vi "MotorControllerGUI.vi"() -> ()   [LabVIEW 2017]
uses:
  device_list.ctl
  device.ctl
  location.ctl
  Newport.CONEXCC.CommandInterface
  <vilib>/Utility/miscctls.llb/LVAnnotationListTypeDef.ctl
  <vilib>/lvdsc/NI_DSC.lvlib
panel:
  out "String":string
  out "Numeric":i32
  in  "Home Y?":bool
  in  "Home X?":bool
  in  "Y COM port":refnum<visa-resource-name>="COM3"
  in  "X COM port":refnum<visa-resource-name>="COM4"
  out "Boolean":bool
  out "error out 2":errorcluster
  in  "Direction Pad":T1={"right+"=FALSE, "right"=FALSE, "left"=FALSE, "left+"=FALSE, "up"=FALSE, "up+"=FALSE, "down+"=FALSE, "down"=FALSE, "motor stop"=FALSE, "Velocity (mm/s)"=2.0, "Step (mm)"=0.1}
  out "Current Location":T2 {"Position"."Position Y" format="%#.3f"; "Position"."Position X" format="%#.3f"}
  out "Key Move?":bool
  out "Center location":T2 {"Position"."Position Y" format="%#.3f"; "Position"."Position X" format="%#.3f"}
  out "Circle":cluster{dbl[], dbl[]}
  in  "Location Description":string="Center"
  in  "Device Description":string="Layout"
  in  "Radius Limit (mm)":dbl=5.0
  out "PA_Set 2":i32
  out "PA_Set":i32
  out "errstring 2":string
  out "errstring":string
  out "error out":errorcluster
  out "X Motor ID":string
  out "Y Motor ID":string
  in  "Delete device":bool
  in  "Device":u16(ring) items=["Layout", "AutoTetherSaver"]
  out "Mouse over item?":bool
  out "Mouse over location":cluster{"X":dbl, "Y":dbl}
  in  "List of default devices":T3 {"List of locations"."Position"."Position Y" format="%#.3f"; "List of locations"."Position"."Position X" format="%#.3f"}
  in  "Load device list":bool
  in  "Default File Path":path
  in  "Add location":bool
  out "Last click location":cluster{"X":dbl, "Y":dbl}
  in  "Rescale location plot":bool caption="Rescale"
  out "Goto Location":T2 {"Position"."Position Y" format="%#.3f"; "Position"."Position X" format="%#.3f"}
  in  "Save device list":bool
  in  "List of devices":T3 {"List of locations"."Position"."Position Y" format="%#.3f"; "List of locations"."Position"."Position X" format="%#.3f"}
  in  "stop":bool
  in  "nSWAT quick move diagram":T5
  out "Location plot":cluster{dbl[], dbl[]}[](graph)
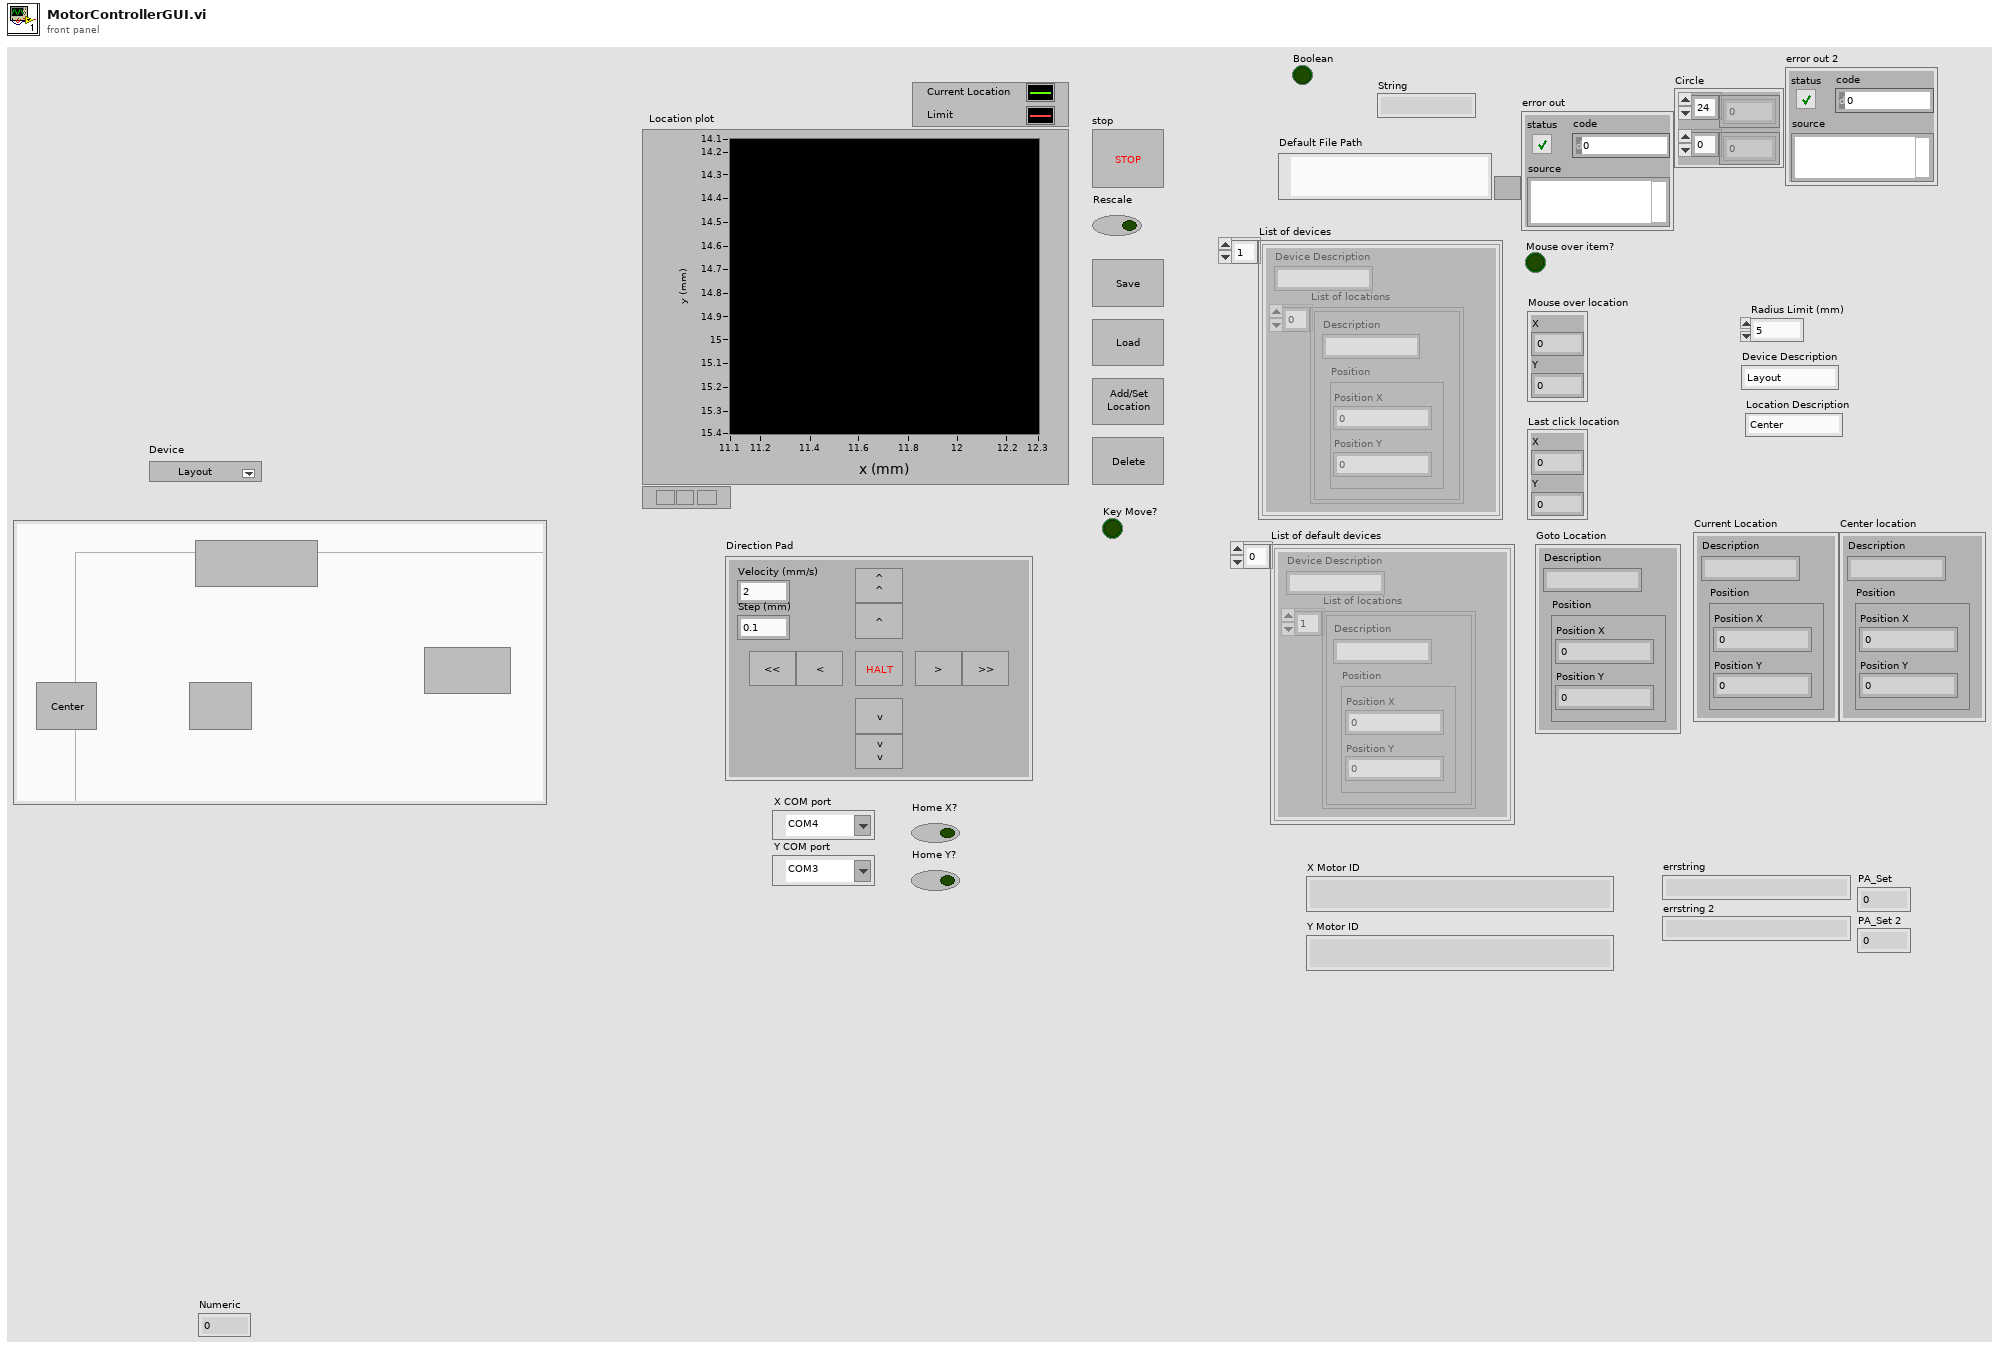
[diagram p1: front panel]
types:
  T1 = cluster{"right+":bool, "right":bool, "left":bool, "left+":bool, "up":bool, "up+":bool, "down+":bool, "down":bool, "motor stop":bool, "Velocity (mm/s)":dbl, "Step (mm)":dbl}
  T2 = typedef "location.ctl" = cluster{"Description":string, "Position":cluster{"Position X":dbl, "Position Y":dbl}}
  T3 = typedef "device_list.ctl" = T4[]
  T4 = typedef "device.ctl" = cluster{"List of locations":T2[], "Device Description":string}
  T5 = cluster{"Button 0":bool, "Button 1":bool, "Button 2":bool, "Button 3":bool}
  T6 = typedef "eventvkey.ctl" = enum16{"ASCII", "Enter", "Return", "Shift", "Ctrl", "Alt", "Cmd", "Opt", "Caps", "NumLock", "Clear", "Break", "Up", "Down", "Left", "Right", "Insert", "Delete", "Home", "End", "PageUp", "PageDown", "Escape", "Help", "Pause", "ScrollLock", "F1", "F2", "F3", "F4", "F5", "F6", "F7", "F8", "F9", "F10", "F11", "F12", "F13", "F14", "F15", "F16", "F17", "F18", "F19", "F20", "F21", "F22", "F23", "F24", "Play", "VolumeUp", "VolumeDown", "Mute", "Two Byte Char"}
  T7 = typedef "LVAnnotationListTypeDef.ctl" = cluster{"Name":string, "Color":u32, "Style":u8, "Point Style":u8, "Name Visible":bool, "Allow Drag":bool, "Annotation Mode":u32, "Plot":i32, "Index":i32, "Position":cluster{"X":dbl, "Y":dbl}, "X Scale":u32, "Y Scale":u32, "Show Arrow":bool, "Lock Name":bool, "Plot Area":i32, "Label Offset":cluster{"X":dbl, "Y":dbl}}[]
  T8 = cluster{"Name":string, "Color":u32, "Style":u8, "Point Style":u8, "Name Visible":bool, "Allow Drag":bool, "Annotation Mode":u32, "Plot":i32, "Index":i32, "Position":cluster{"X":dbl, "Y":dbl}, "X Scale":u32, "Y Scale":u32, "Show Arrow":bool, "Lock Name":bool, "Plot Area":i32, "Label Offset":cluster{"X":dbl, "Y":dbl}}
  T9 = typedef "LVPoint32TypeDef.ctl" = cluster{"Horizontal":i32, "Vertical":i32}
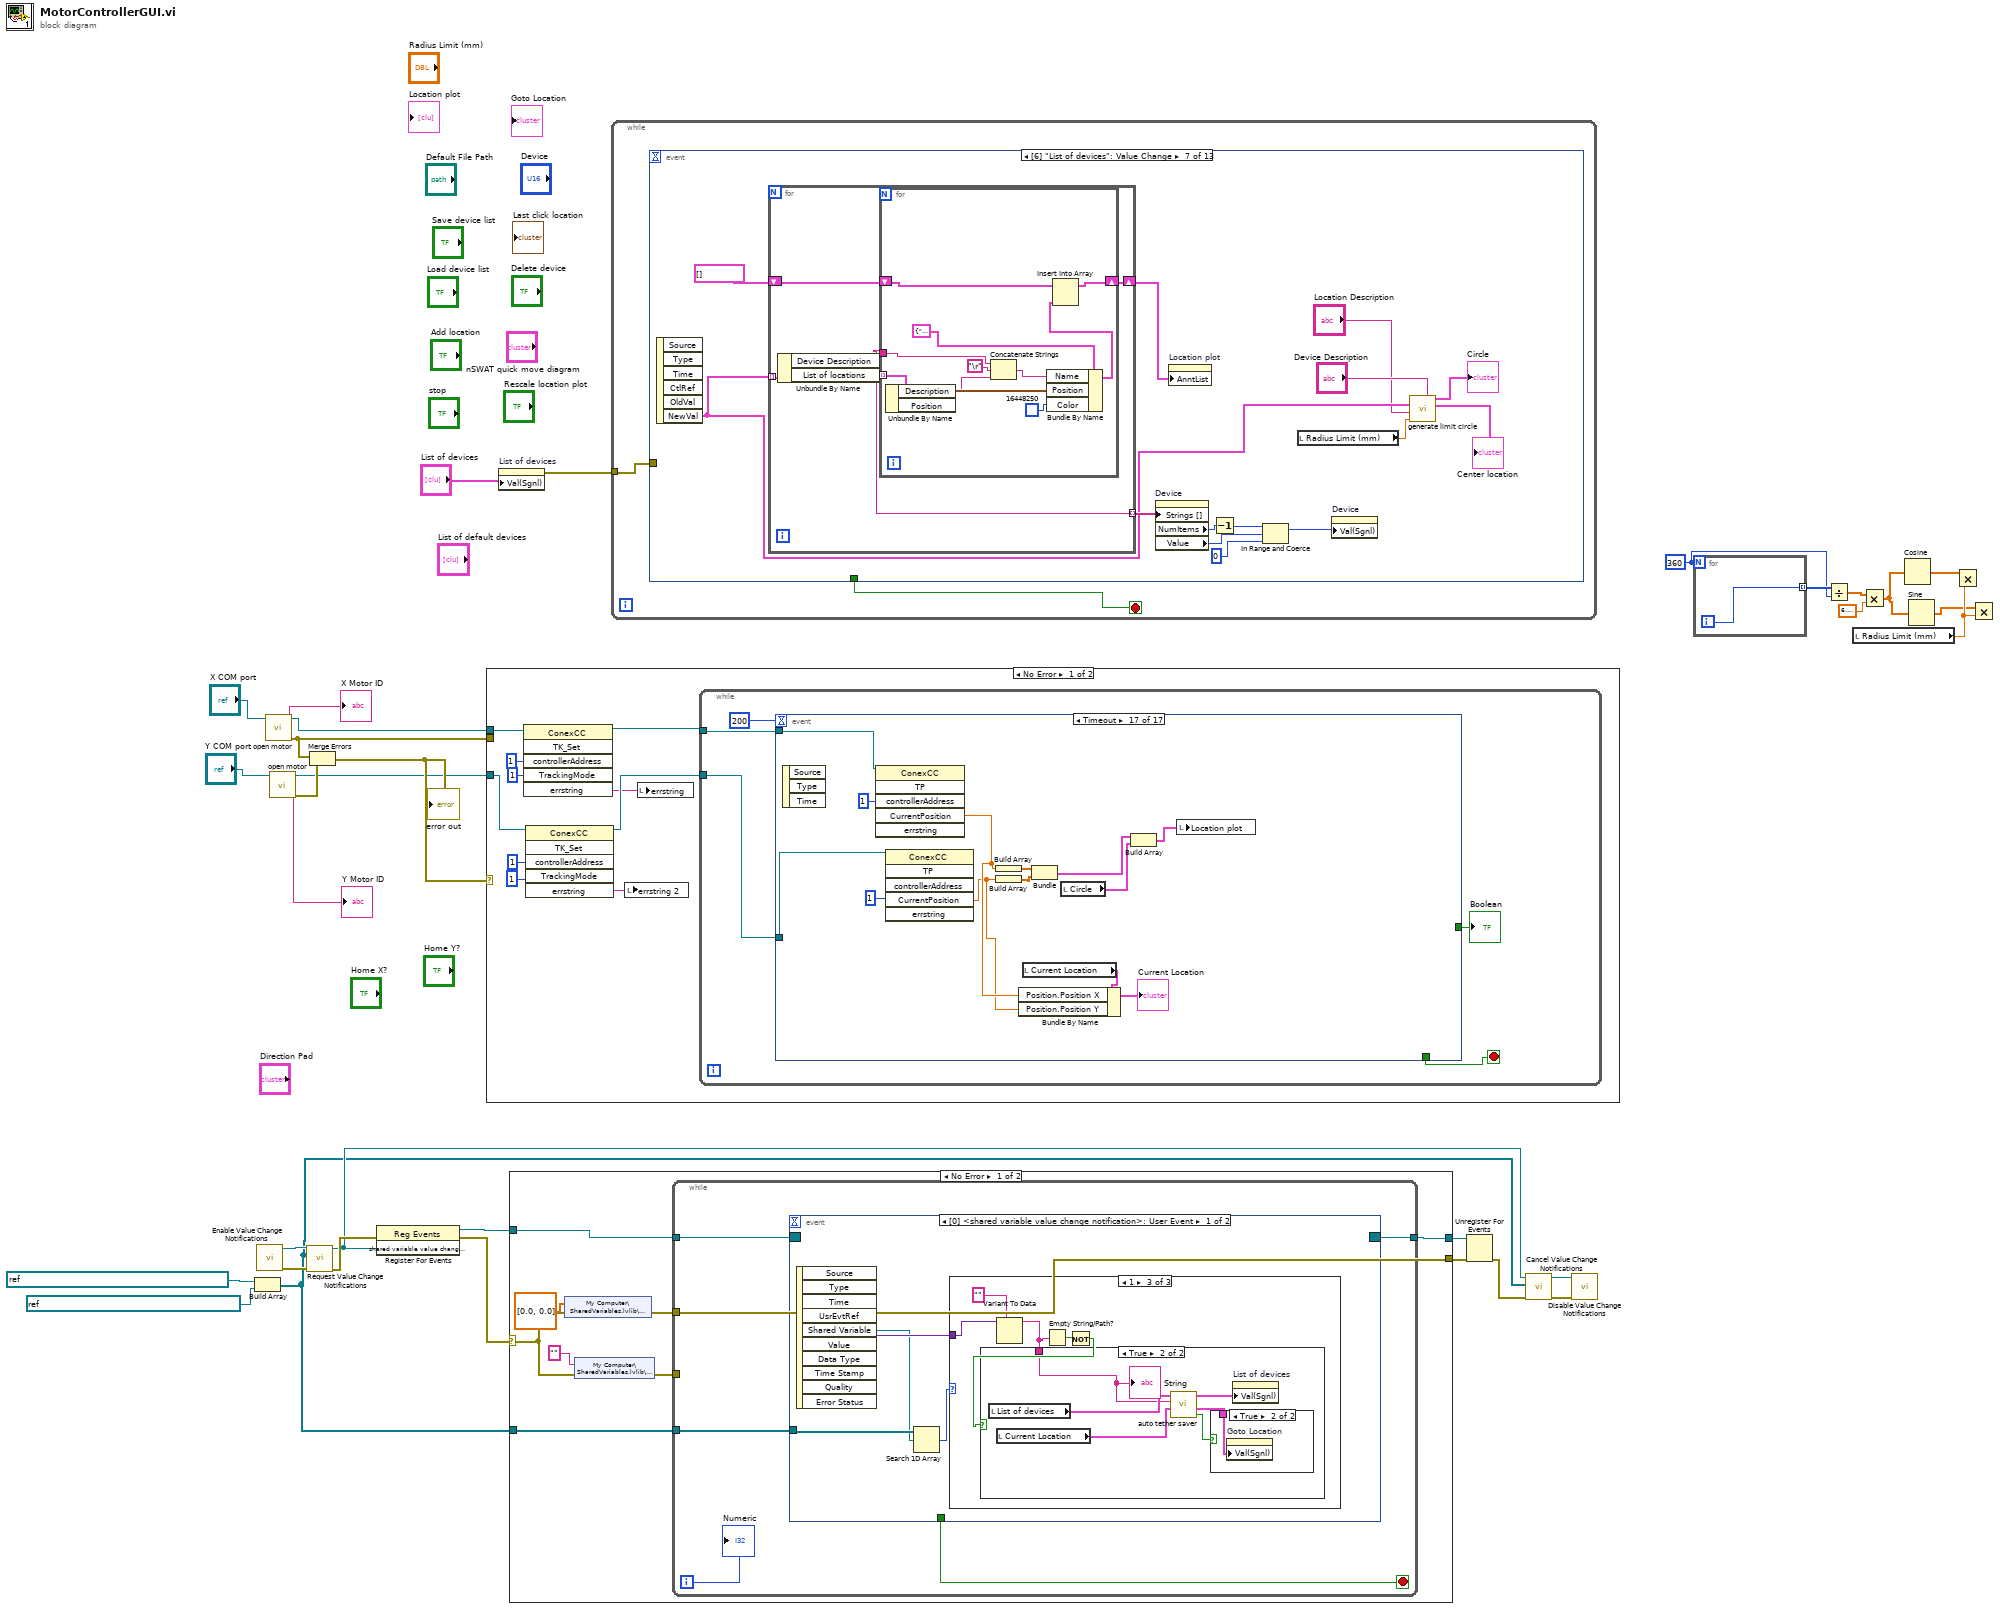
[diagram p0: block diagram]
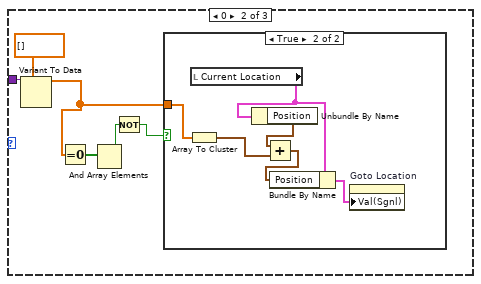
[diagram p3: hidden frame]
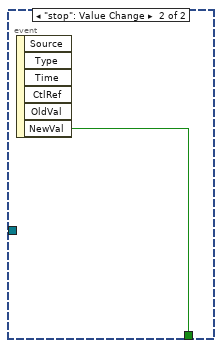
[diagram p7: hidden frame]
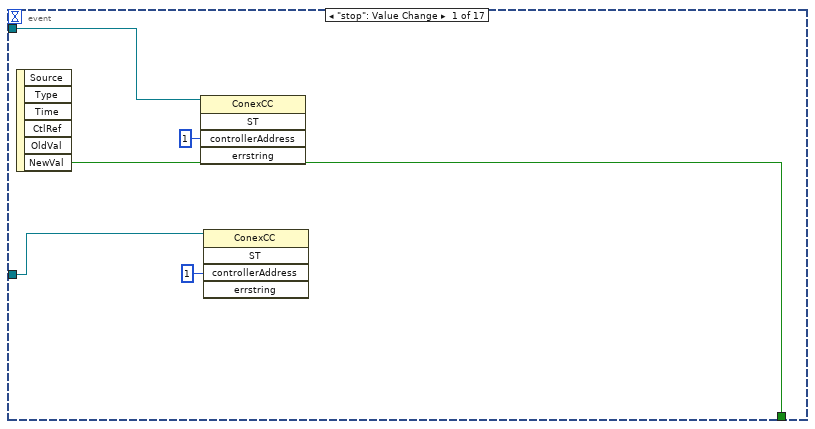
[diagram p9: hidden frame]
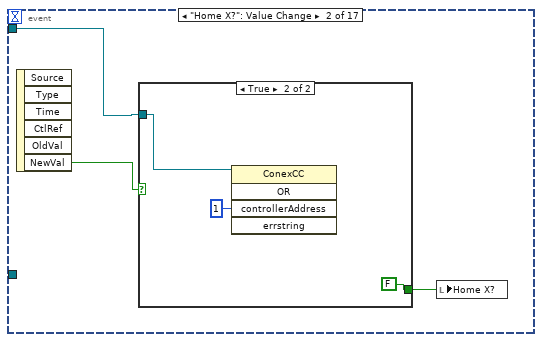
[diagram p10: hidden frame]
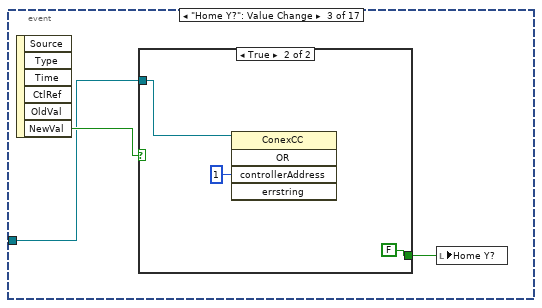
[diagram p12: hidden frame]
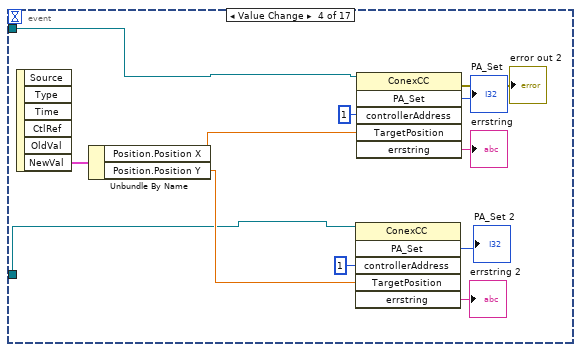
[diagram p14: hidden frame]
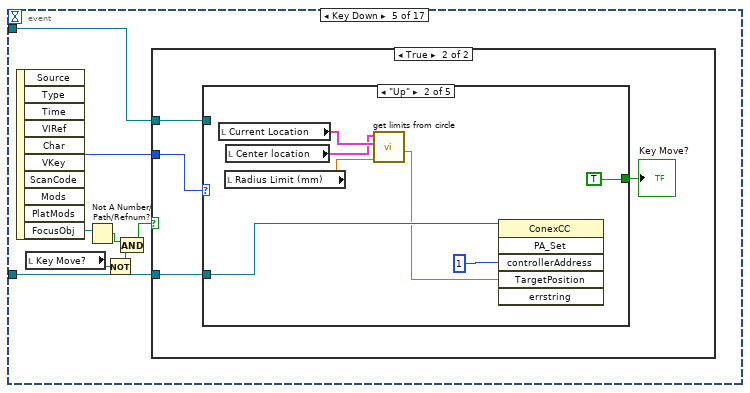
[diagram p15: hidden frame]
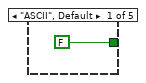
[diagram p17: hidden frame]
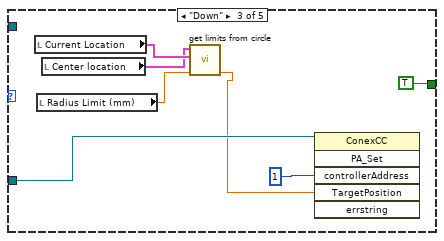
[diagram p18: hidden frame]
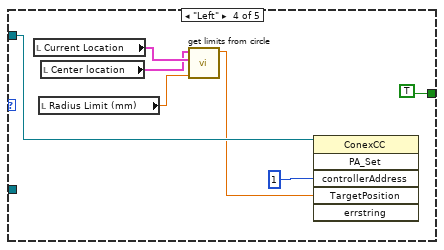
[diagram p19: hidden frame]
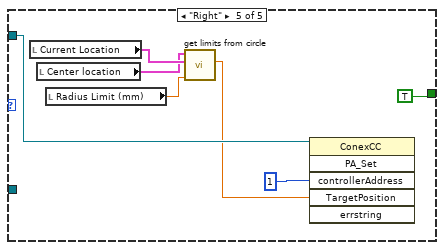
[diagram p20: hidden frame]
diagram:
  w17 = 360
  n1 = Build Array(refnum<k21> "\\\\My Computer\\SharedVariables\\ImageClick" ("Project Variable Control"), refnum<k21> "\\\\My Computer\\SharedVariables\\TraceInfo" ("Project Variable Control")) -> (w2:refnum<k21>[])
  n2 = call <vilib>:"Enable Value Change Notifications.vi"() -> ("error out"=w13:errorcluster, "shared variable value change notification"=w14:refnum<user-event>)  [unwired: 10 in]
  n3 = call "open motor.vi"("COM port"="X COM port") -> ("error out"=w28:errorcluster, "Motor ID"=→"X Motor ID":string, "CONEX_CC"=w27:refnum<k24>)  [unwired: 8 in]
  n4 = call "open motor.vi"("COM port"="Y COM port") -> ("error out"=w30:errorcluster, "Motor ID"=→"Y Motor ID":string, "CONEX_CC"=w26:refnum<k24>)  [unwired: 8 in]
  n5 = call <vilib>:"Request Value Change Notifications.vi"("error in (no error)"=w13, "shared variables"=w2, "notification refnum"=w14) -> ("error out"=w12:errorcluster, "shared variable value change notification"=w6:refnum<user-event>)  [unwired: 6 in, 1 out]
  n6 = Merge Errors(w28, w30) -> (w29:errorcluster)
  "error out" <- w29
  n7 = register-events(error in=w12, w6) -> (reference out=w11:refnum<event-registration>, error out=w5:errorcluster)  [unwired: 1 in]
  n8 = case shown="No Error" w29 {
    tunnel: w28 -> [_ _]
    tunnel: w27 -> [w37 _]
    tunnel: w26 -> [w41 _]
    frame No Error {
      n9 = invoke class="ConexCC" method="TK_Set"(reference=w37, "controllerAddress"=1, "TrackingMode"=1) -> (reference out=w36:refnum<k24>, "errstring"=w35:string)  [unwired: 3 in, 4 out]
      n10 = invoke class="ConexCC" method="TK_Set"(reference=w41, "controllerAddress"=1, "TrackingMode"=1) -> (reference out=w40:refnum<k24>, "errstring"=w34:string)  [unwired: 3 in, 4 out]
      n11 = local write "errstring 2"(w34) -> ()
      n12 = local write "errstring"(w35) -> ()
      n13 = while {
        tunnel: w36 -> [w48]
        tunnel: w40 -> [w47]
        stop <- w45 stop-if-true
        n14 = event shown="[16] Timeout" {
          selector: _ -> [_ _ _ _ _ _ _ _ _ _ _ _ _ _ _ _ _]
          dyn-events: _ -> [_ _ _ _ _ _ _ _ _ _ _ _ _ _ _ _ _]
          timeout: 200 -> [_ _ _ _ _ _ _ _ _ _ _ _ _ _ _ _ _]
          tunnel: [w53 _ _ _ _ _ _ _ _ _ _ _ _ _ _ _ _] -> w45
          tunnel: w48 -> [w50 w55 _ w68 w83 w127 w130 w138 _ _ w167 w177 _ _ w224 w242 w271]
          tunnel: w47 -> [w49 _ w60 w67 w82 w126 w129 w137 w147 w157 _ _ w188 w206 _ _ w270]
          tunnel: [_ _ _ _ _ _ _ _ _ _ _ _ w187 w205 w223 w241 _] -> w44
          event "stop": Value Change {
            n15 = event-data() -> ("NewVal"=w53:bool)  [unwired: 1 in, 5 out]
            n16 = invoke class="ConexCC" method="ST"(reference=w50, "controllerAddress"=1) -> ()  [unwired: 3 in, 5 out]
            n17 = invoke class="ConexCC" method="ST"(reference=w49, "controllerAddress"=1) -> ()  [unwired: 3 in, 5 out]
          }
          event "Home X?": Value Change {
            n18 = event-data() -> ("NewVal"=w56:bool)  [unwired: 1 in, 5 out]
            n19 = case shown="True" w56 {
              tunnel: w55 -> [_ w59]
              tunnel: [_ FALSE ("Home X?")] -> w54
              frame False {
              }
              frame True {
                n20 = invoke class="ConexCC" method="OR"(reference=w59, "controllerAddress"=1) -> ()  [unwired: 3 in, 5 out]
              }
            }
            n21 = local write "Home X?"(w54) -> ()
          }
          event "Home Y?": Value Change {
            n22 = event-data() -> ("NewVal"=w62:bool)  [unwired: 1 in, 5 out]
            n23 = case shown="True" w62 {
              tunnel: w60 -> [_ w65]
              tunnel: [_ FALSE ("Home X?")] -> w61
              frame False {
              }
              frame True {
                n24 = invoke class="ConexCC" method="OR"(reference=w65, "controllerAddress"=1) -> ()  [unwired: 3 in, 5 out]
              }
            }
            n25 = local write "Home Y?"(w61) -> ()
          }
          event Value Change {
            n26 = event-data() -> ("NewVal"=w77:T2)  [unwired: 1 in, 5 out]
            n27 = Unbundle By Name(w77) -> ("Position.Position X"=w76:dbl, "Position.Position Y"=w75:dbl)
            n28 = invoke class="ConexCC" method="PA_Set"(reference=w67, "controllerAddress"=1, "TargetPosition"=w75) -> ("PA_Set"=→"PA_Set 2":i32, "errstring"=→"errstring 2":string)  [unwired: 3 in, 4 out]
            n29 = invoke class="ConexCC" method="PA_Set"(reference=w68, "controllerAddress"=1, "TargetPosition"=w76) -> (error out=→"error out 2":errorcluster, "PA_Set"=→"PA_Set":i32, "errstring"=→"errstring":string)  [unwired: 3 in, 3 out]
          }
          event Key Down {
            n30 = event-data() -> ("VKey"=w84:T6, "FocusObj"=w85:refnum<vi>)  [unwired: 1 in, 8 out]
            n31 = local read "Key Move?"() -> (w80:bool)
            n32 = Not A Number/Path/Refnum?(number/path/refnum=w85) -> (NaN/Path/Refnum?=w81:bool)
            n33 = Not(x=w80) -> (.not. x?=w79:bool)
            n34 = And(x=w81, y=w79) -> (x .and. y?=w78:bool)
            n35 = case shown="True" w78 {
              tunnel: w84 -> [_ w89]
              tunnel: w83 -> [_ w87]
              tunnel: w82 -> [_ w86]
              frame False {
              }
              frame True {
                n36 = case shown="\"Up\"" w89 {
                  tunnel: [FALSE TRUE TRUE TRUE TRUE] -> w88
                  tunnel: w87 -> [_ _ _ w107 w114]
                  tunnel: w86 -> [_ w96 w100 _ _]
                  frame "ASCII", Default {
                  }
                  frame "Up" {
                    n37 = local read "Current Location"() -> (w94:T2)
                    n38 = local read "Radius Limit (mm)"() -> (w92:dbl)
                    n39 = local read "Center location"() -> (w93:T2)
                    n40 = call "get limits from circle.vi"("Radius"=w92, "Current Location"=w94, "Center location"=w93) -> ("Ymin given x"=w91:dbl)  [unwired: 5 in, 3 out]
                    n41 = invoke class="ConexCC" method="PA_Set"(reference=w96, "controllerAddress"=1, "TargetPosition"=w91) -> ()  [unwired: 3 in, 6 out]
                  }
                  frame "Down" {
                    n42 = local read "Current Location"() -> (w102:T2)
                    n43 = local read "Radius Limit (mm)"() -> (w99:dbl)
                    n44 = local read "Center location"() -> (w101:T2)
                    n45 = call "get limits from circle.vi"("Radius"=w99, "Current Location"=w102, "Center location"=w101) -> ("Ymax given x"=w98:dbl)  [unwired: 5 in, 3 out]
                    n46 = invoke class="ConexCC" method="PA_Set"(reference=w100, "controllerAddress"=1, "TargetPosition"=w98) -> ()  [unwired: 3 in, 6 out]
                  }
                  frame "Left" {
                    n47 = local read "Current Location"() -> (w109:T2)
                    n48 = local read "Radius Limit (mm)"() -> (w105:dbl)
                    n49 = local read "Center location"() -> (w108:T2)
                    n50 = call "get limits from circle.vi"("Radius"=w105, "Current Location"=w109, "Center location"=w108) -> ("Xmin given y"=w106:dbl)  [unwired: 5 in, 3 out]
                    n51 = invoke class="ConexCC" method="PA_Set"(reference=w107, "controllerAddress"=1, "TargetPosition"=w106) -> ()  [unwired: 3 in, 6 out]
                  }
                  frame "Right" {
                    n52 = local read "Current Location"() -> (w116:T2)
                    n53 = local read "Center location"() -> (w115:T2)
                    n54 = local read "Radius Limit (mm)"() -> (w113:dbl)
                    n55 = call "get limits from circle.vi"("Radius"=w113, "Current Location"=w116, "Center location"=w115) -> ("Xmax given y"=w112:dbl)  [unwired: 5 in, 3 out]
                    n56 = invoke class="ConexCC" method="PA_Set"(reference=w114, "controllerAddress"=1, "TargetPosition"=w112) -> ()  [unwired: 3 in, 6 out]
                  }
                }
                "Key Move?" <- w88
              }
            }
          }
          event "Direction Pad.Velocity (mm/s)": Value Change {
            w119 = 1 ("controllerAddress")
            n57 = event-data() -> ("NewVal"=w125:dbl)  [unwired: 1 in, 5 out]
            n58 = invoke class="ConexCC" method="VA_Set"(reference=w126, "controllerAddress"=1, "Velocity"=w125) -> ()  [unwired: 3 in, 6 out]
            n59 = invoke class="ConexCC" method="VA_Set"(reference=w127, "controllerAddress"=w119, "Velocity"=w125) -> (reference out=w123:refnum<k24>)  [unwired: 3 in, 5 out]
            n60 = invoke class="ConexCC" method="VA_Get"(reference=w123, "controllerAddress"=w119) -> ("Velocity"=w121:dbl)  [unwired: 4 in, 5 out]
            n61 = local read "Direction Pad"() -> (w122:T1)
            n62 = in-place {
              in-place-border: w121 -> [w128]
              n63 = in-place-cluster #1(w122) -> ()  [unwired: 1 out]
              n64 = in-place-cluster #1("Velocity (mm/s)"=w128) -> (w120:T1)
            }
            n65 = local write "Direction Pad"(w120) -> ()
          }
          event Key Up {
            n66 = event-data() -> ()  [unwired: 1 in, 8 out]
            n67 = local read "Key Move?"() -> (w131:bool)
            n68 = case shown="True" w131 {
              tunnel: w130 -> [_ w136]
              tunnel: w129 -> [_ w134]
              frame False {
              }
              frame True {
                n69 = invoke class="ConexCC" method="ST"(reference=w136, "controllerAddress"=1) -> ()  [unwired: 3 in, 5 out]
                n70 = invoke class="ConexCC" method="ST"(reference=w134, "controllerAddress"=1) -> ()  [unwired: 3 in, 5 out]
                n71 = local write "Key Move?"(FALSE ("Key Move?")) -> ()
              }
            }
          }
          event "Direction Pad.motor stop": Value Change {
            n72 = event-data() -> ("NewVal"=w139:bool)  [unwired: 1 in, 5 out]
            n73 = case shown="True" w139 {
              tunnel: w138 -> [_ w145]
              tunnel: w137 -> [_ w144]
              frame False {
              }
              frame True {
                n74 = invoke class="ConexCC" method="ST"(reference=w145, "controllerAddress"=1) -> ()  [unwired: 3 in, 5 out]
                n75 = invoke class="ConexCC" method="ST"(reference=w144, "controllerAddress"=1) -> ()  [unwired: 3 in, 5 out]
                n76 = local read "Direction Pad"() -> (w141:T1)
                n77 = in-place {
                  n78 = in-place-cluster #2(w141) -> ()  [unwired: 1 out]
                  n79 = in-place-cluster #2("motor stop"=FALSE) -> (w140:T1)
                }
                n80 = local write "Direction Pad"(w140) -> ()
              }
            }
          }
          event "Direction Pad.up+": Value Change {
            n81 = event-data() -> ("NewVal"=w148:bool)  [unwired: 1 in, 5 out]
            n82 = case shown="True" w148 {
              tunnel: w147 -> [w149 w152]
              frame False {
                n83 = invoke class="ConexCC" method="ST"(reference=w149, "controllerAddress"=1) -> ()  [unwired: 3 in, 5 out]
              }
              frame True {
                n84 = local read "Current Location"() -> (w156:T2)
                n85 = local read "Radius Limit (mm)"() -> (w154:dbl)
                n86 = local read "Center location"() -> (w155:T2)
                n87 = call "get limits from circle.vi"("Radius"=w154, "Current Location"=w156, "Center location"=w155) -> ("Ymin given x"=w151:dbl)  [unwired: 5 in, 3 out]
                n88 = invoke class="ConexCC" method="PA_Set"(reference=w152, "controllerAddress"=1, "TargetPosition"=w151) -> ()  [unwired: 3 in, 6 out]
              }
            }
          }
          event "Direction Pad.down+": Value Change {
            n89 = event-data() -> ("NewVal"=w158:bool)  [unwired: 1 in, 5 out]
            n90 = case shown="True" w158 {
              tunnel: w157 -> [w159 w162]
              frame False {
                n91 = invoke class="ConexCC" method="ST"(reference=w159, "controllerAddress"=1) -> ()  [unwired: 3 in, 5 out]
              }
              frame True {
                n92 = local read "Current Location"() -> (w166:T2)
                n93 = local read "Radius Limit (mm)"() -> (w164:dbl)
                n94 = local read "Center location"() -> (w165:T2)
                n95 = call "get limits from circle.vi"("Radius"=w164, "Current Location"=w166, "Center location"=w165) -> ("Ymax given x"=w161:dbl)  [unwired: 5 in, 3 out]
                n96 = invoke class="ConexCC" method="PA_Set"(reference=w162, "controllerAddress"=1, "TargetPosition"=w161) -> ()  [unwired: 3 in, 6 out]
              }
            }
          }
          event "Direction Pad.left+": Value Change {
            n97 = event-data() -> ("NewVal"=w168:bool)  [unwired: 1 in, 5 out]
            n98 = case shown="False" w168 {
              tunnel: w167 -> [w169 w172]
              frame False {
                n99 = invoke class="ConexCC" method="ST"(reference=w169, "controllerAddress"=1) -> ()  [unwired: 3 in, 5 out]
              }
              frame True {
                n100 = local read "Current Location"() -> (w176:T2)
                n101 = local read "Radius Limit (mm)"() -> (w174:dbl)
                n102 = local read "Center location"() -> (w175:T2)
                n103 = call "get limits from circle.vi"("Radius"=w174, "Current Location"=w176, "Center location"=w175) -> ("Xmin given y"=w171:dbl)  [unwired: 5 in, 3 out]
                n104 = invoke class="ConexCC" method="PA_Set"(reference=w172, "controllerAddress"=1, "TargetPosition"=w171) -> ()  [unwired: 3 in, 6 out]
              }
            }
          }
          event "Direction Pad.right+": Value Change {
            n105 = event-data() -> ("NewVal"=w178:bool)  [unwired: 1 in, 5 out]
            n106 = case shown="True" w178 {
              tunnel: w177 -> [w179 w182]
              frame False {
                n107 = invoke class="ConexCC" method="ST"(reference=w179, "controllerAddress"=1) -> ()  [unwired: 3 in, 5 out]
              }
              frame True {
                n108 = local read "Current Location"() -> (w186:T2)
                n109 = local read "Radius Limit (mm)"() -> (w184:dbl)
                n110 = local read "Center location"() -> (w185:T2)
                n111 = call "get limits from circle.vi"("Radius"=w184, "Current Location"=w186, "Center location"=w185) -> ("Xmax given y"=w181:dbl)  [unwired: 5 in, 3 out]
                n112 = invoke class="ConexCC" method="PA_Set"(reference=w182, "controllerAddress"=1, "TargetPosition"=w181) -> ()  [unwired: 3 in, 6 out]
              }
            }
          }
          event "Direction Pad.up": Value Change {
            n113 = event-data() -> ("NewVal"=w189:bool)  [unwired: 1 in, 5 out]
            n114 = case shown="True" w189 {
              tunnel: w188 -> [_ w200]
              tunnel: [_ w190] -> w187
              frame False {
              }
              frame True {
                n115 = local read "Current Location"() -> (w201:T2)
                n116 = local read "Radius Limit (mm)"() -> (w202:dbl)
                n117 = local read "Center location"() -> (w203:T2)
                n118 = local read "Direction Pad"() -> (w197:T1)
                n119 = Unbundle By Name(w201) -> ("Position.Position Y"=w199:dbl)
                n120 = Unbundle By Name(w197) -> ("Step (mm)"=w196:dbl)
                n121 = in-place {
                  n122 = in-place-cluster #3(w197) -> ()  [unwired: 1 out]
                  n123 = in-place-cluster #3("up"=FALSE ("motor stop")) -> (w198:T1)
                }
                n124 = call "get limits from circle.vi"("Radius"=w202, "Current Location"=w201, "Center location"=w203) -> ("Ymax given x"=w192:dbl, "Ymin given x"=w193:dbl)  [unwired: 5 in, 2 out]
                n125 = Subtract(x=w199, y=w196) -> (x-y=w194:dbl)
                n126 = In Range and Coerce(upper limit=w192, x=w194, lower limit=w193) -> (coerced(x)=w191:dbl, In Range?=w190:bool)
                n127 = local write "Direction Pad"(w198) -> ()
                n128 = invoke class="ConexCC" method="PA_Set"(reference=w200, "controllerAddress"=1, "TargetPosition"=w191) -> ()  [unwired: 3 in, 6 out]
              }
            }
          }
          event "Direction Pad.down": Value Change {
            n129 = event-data() -> ("NewVal"=w207:bool)  [unwired: 1 in, 5 out]
            n130 = case shown="True" w207 {
              tunnel: w206 -> [_ w218]
              tunnel: [_ w208] -> w205
              frame False {
              }
              frame True {
                n131 = local read "Current Location"() -> (w219:T2)
                n132 = local read "Radius Limit (mm)"() -> (w220:dbl)
                n133 = local read "Center location"() -> (w221:T2)
                n134 = local read "Direction Pad"() -> (w215:T1)
                n135 = Unbundle By Name(w219) -> ("Position.Position Y"=w217:dbl)
                n136 = Unbundle By Name(w215) -> ("Step (mm)"=w214:dbl)
                n137 = in-place {
                  n138 = in-place-cluster #4(w215) -> ()  [unwired: 1 out]
                  n139 = in-place-cluster #4("down"=FALSE ("motor stop")) -> (w216:T1)
                }
                n140 = call "get limits from circle.vi"("Radius"=w220, "Current Location"=w219, "Center location"=w221) -> ("Ymax given x"=w210:dbl, "Ymin given x"=w211:dbl)  [unwired: 5 in, 2 out]
                n141 = Add(x=w217, y=w214) -> (x+y=w212:dbl)
                n142 = In Range and Coerce(upper limit=w210, x=w212, lower limit=w211) -> (coerced(x)=w209:dbl, In Range?=w208:bool)
                n143 = local write "Direction Pad"(w216) -> ()
                n144 = invoke class="ConexCC" method="PA_Set"(reference=w218, "controllerAddress"=1, "TargetPosition"=w209) -> ()  [unwired: 3 in, 6 out]
              }
            }
          }
          event "Direction Pad.left": Value Change {
            n145 = event-data() -> ("NewVal"=w225:bool)  [unwired: 1 in, 5 out]
            n146 = case shown="True" w225 {
              tunnel: w224 -> [_ w236]
              tunnel: [_ w226] -> w223
              frame False {
              }
              frame True {
                n147 = local read "Current Location"() -> (w237:T2)
                n148 = local read "Radius Limit (mm)"() -> (w238:dbl)
                n149 = local read "Center location"() -> (w239:T2)
                n150 = local read "Direction Pad"() -> (w234:T1)
                n151 = Unbundle By Name(w237) -> ("Position.Position X"=w227:dbl)
                n152 = Unbundle By Name(w234) -> ("Step (mm)"=w233:dbl)
                n153 = in-place {
                  n154 = in-place-cluster #5(w234) -> ()  [unwired: 1 out]
                  n155 = in-place-cluster #5("left"=FALSE ("motor stop")) -> (w235:T1)
                }
                n156 = call "get limits from circle.vi"("Radius"=w238, "Current Location"=w237, "Center location"=w239) -> ("Xmax given y"=w228:dbl, "Xmin given y"=w229:dbl)  [unwired: 5 in, 2 out]
                n157 = Subtract(x=w227, y=w233) -> (x-y=w231:dbl)
                n158 = In Range and Coerce(upper limit=w228, x=w231, lower limit=w229) -> (coerced(x)=w230:dbl, In Range?=w226:bool)
                n159 = local write "Direction Pad"(w235) -> ()
                n160 = invoke class="ConexCC" method="PA_Set"(reference=w236, "controllerAddress"=1, "TargetPosition"=w230) -> ()  [unwired: 3 in, 6 out]
              }
            }
          }
          event "Direction Pad.right": Value Change {
            n161 = event-data() -> ("NewVal"=w243:bool)  [unwired: 1 in, 5 out]
            n162 = case shown="True" w243 {
              tunnel: w242 -> [_ w254]
              tunnel: [_ w244] -> w241
              frame False {
              }
              frame True {
                n163 = local read "Current Location"() -> (w255:T2)
                n164 = local read "Radius Limit (mm)"() -> (w256:dbl)
                n165 = local read "Center location"() -> (w257:T2)
                n166 = local read "Direction Pad"() -> (w252:T1)
                n167 = Unbundle By Name(w255) -> ("Position.Position X"=w245:dbl)
                n168 = Unbundle By Name(w252) -> ("Step (mm)"=w251:dbl)
                n169 = in-place {
                  n170 = in-place-cluster #6(w252) -> ()  [unwired: 1 out]
                  n171 = in-place-cluster #6("right"=FALSE ("motor stop")) -> (w253:T1)
                }
                n172 = call "get limits from circle.vi"("Radius"=w256, "Current Location"=w255, "Center location"=w257) -> ("Xmax given y"=w246:dbl, "Xmin given y"=w247:dbl)  [unwired: 5 in, 2 out]
                n173 = Add(x=w245, y=w251) -> (x+y=w249:dbl)
                n174 = In Range and Coerce(upper limit=w246, x=w249, lower limit=w247) -> (coerced(x)=w248:dbl, In Range?=w244:bool)
                n175 = local write "Direction Pad"(w253) -> ()
                n176 = invoke class="ConexCC" method="PA_Set"(reference=w254, "controllerAddress"=1, "TargetPosition"=w248) -> ()  [unwired: 3 in, 6 out]
              }
            }
          }
          event Timeout {
            n177 = event-data() -> ()  [unwired: 1 in, 3 out]
            n178 = invoke class="ConexCC" method="TP"(reference=w271, "controllerAddress"=1) -> ("CurrentPosition"=w260:dbl)  [unwired: 4 in, 5 out]
            n179 = invoke class="ConexCC" method="TP"(reference=w270, "controllerAddress"=1) -> ("CurrentPosition"=w259:dbl)  [unwired: 4 in, 5 out]
            n180 = Build Array(w260) -> (w266:dbl[])
            n181 = Build Array(w259) -> (w267:dbl[])
            n182 = local read "Current Location"() -> (w261:T2)
            n183 = Bundle By Name(cluster=w261, "Position.Position X"=w260, "Position.Position Y"=w259) -> (→"Current Location":T2)
            n184 = Bundle(w266, w267) -> (w265:cluster{dbl[], dbl[]})  [unwired: 1 in]
            n185 = local read "Circle"() -> (w263:cluster{dbl[], dbl[]})
            n186 = Build Array(w265, w263) -> (w264:cluster{dbl[], dbl[]}[])
            n187 = local write "Location plot"(w264) -> ()
          }
        }
        "Boolean" <- w44
      }
    }
    frame Error {
    }
  }
  n188 = property on="List of devices" class="Arr (strict)"("Val(Sgnl)"="List of devices") -> (error out=w33:errorcluster)  [unwired: 2 in, 1 out]
  n189 = case shown="No Error" w5 {
    selector: w5 -> [w273 w315]
    tunnel: w11 -> [w279 w314]
    tunnel: [w278 w314] -> w10
    tunnel: [w277 w315] -> w4
    tunnel: w2 -> [w275 _]
    frame No Error {
      n190 = shared-variable "My Computer\\SharedVariables.lvlib\\ImageClick"(dbl[] [0.0, 0.0] ("ImageClick"), error in=w273) -> (error out=w277:errorcluster)
      n191 = shared-variable "My Computer\\SharedVariables.lvlib\\TraceInfo"("", error in=w273) -> (error out=w272:errorcluster)
      n192 = while {
        tunnel: w279 -> [w283]
        tunnel: [w282] -> w278
        tunnel: w277 -> [_]
        tunnel: w275 -> [w280]
        tunnel: w272 -> [_]
        i -> [w284]
        stop <- w281 stop-if-true
        n193 = event shown="[0] <shared variable value change notification>: User Event" {
          selector: w283 -> [_ _]
          dyn-events: [_ _] -> w282
          timeout: _ -> [_ _]
          tunnel: [_ w313] -> w281
          tunnel: w280 -> [w287 _]
          event User Event {
            n194 = event-data() -> ("Shared Variable"=w285:refnum<k21>, "Value"=w288:variant)  [unwired: 1 in, 8 out]
            n195 = Search 1D Array(1D array=w287, element=w285) -> (index of element=w286:i32)  [unwired: 1 in]
            n196 = case shown="1" w286 {
              tunnel: w288 -> [_ w294 w305]
              frame -1, Default {
              }
              frame 0 {
                n197 = Variant To Data(type=dbl[] [], Variant=w294) -> (data=w292:dbl[])  [unwired: 1 in, 1 out]
                n198 = Equal To 0?(x=w292) -> (x = 0?=w291:bool[])
                n199 = And Array Elements(Boolean array=w291) -> (logical AND=w290:bool)
                n200 = Not(x=w290) -> (.not. x?=w289:bool)
                n201 = case shown="True" w289 {
                  tunnel: w292 -> [_ w300]
                  frame False {
                  }
                  frame True {
                    n202 = Array To Cluster(array=w300) -> (cluster=w297:cluster{"[0]":dbl, "[1]":dbl})
                    n203 = local read "Current Location"() -> (w299:T2)
                    n204 = Unbundle By Name(w299) -> ("Position"=w298:cluster{"Position X":dbl, "Position Y":dbl})
                    n205 = Add(x=w298, y=w297) -> (x+y=w296:cluster{dbl, dbl})
                    n206 = Bundle By Name(cluster=w299, "Position"=w296) -> (w295:T2)
                    n207 = property on="Goto Location" class="Clust (strict)"("Val(Sgnl)"=w295) -> ()  [unwired: 2 in, 2 out]
                  }
                }
              }
              frame 1 {
                n208 = Variant To Data(type="", Variant=w305) -> (data=w303:string)  [unwired: 1 in, 1 out]
                n209 = Empty String/Path?(string/path=w303) -> (empty?=w302:bool)
                n210 = Not(x=w302) -> (.not. x?=w301:bool)
                n211 = case shown="True" w301 {
                  tunnel: w303 -> [_ w310]
                  frame False {
                  }
                  frame True {
                    n212 = local read "List of devices"() -> (w311:T3)
                    n213 = local read "Current Location"() -> (w309:T2)
                    n214 = call "auto tether saver.vi"("Current Location"=w309, "TraceName"=w310, "List of devices"=w311) -> ("Found?"=w308:bool, "Location of input"=w307:T2, "List of devices 2"=w306:T3)  [unwired: 6 in]
                    n215 = case shown="True" w308 {
                      tunnel: w307 -> [_ w312]
                      frame False {
                      }
                      frame True {
                        n216 = property on="Goto Location" class="Clust (strict)"("Val(Sgnl)"=w312) -> ()  [unwired: 2 in, 2 out]
                      }
                    }
                    n217 = property on="List of devices" class="Arr (strict)"("Val(Sgnl)"=w306) -> ()  [unwired: 2 in, 2 out]
                    "String" <- w310
                  }
                }
              }
            }
          }
          event "stop": Value Change {
            n218 = event-data() -> ("NewVal"=w313:bool)  [unwired: 1 in, 5 out]
          }
        }
        "Numeric" <- w284
      }
    }
    frame Error {
    }
  }
  n219 = while {
    tunnel: w33 -> [w316]
    stop <- w317 stop-if-true
    n220 = event shown="[6] \"List of devices\": Value Change" {
      selector: _ -> [_ _ _ _ _ _ _ _ _ _ _ _ _]
      dyn-events: _ -> [_ _ _ _ _ _ _ _ _ _ _ _ _]
      timeout: _ -> [_ _ _ _ _ _ _ _ _ _ _ _ _]
      tunnel: [w318 _ _ _ _ _ _ _ _ _ _ _ _] -> w317
      tunnel: w316 -> [_ _ _ _ _ _ _ _ _ _ _ _ _]
      event "stop": Value Change {
        n221 = event-data() -> ("NewVal"=w318:bool)  [unwired: 1 in, 5 out]
      }
      event "nSWAT quick move diagram": Value Change {
        n222 = event-data() -> ("OldVal"=w319:T5, "NewVal"=w323:T5)  [unwired: 1 in, 4 out]
        n223 = local write "nSWAT quick move diagram"(w319) -> ()
        n224 = Cluster To Array(cluster=w323) -> (array=w322:bool[])
        n225 = for {
          tunnel: w322 -> [w337] mode=indexing
          tunnel: [w337] -> w321
          tunnel: [w336] -> w320
          i -> [w336]
          stop <- w337 stop-if-true
        }
        n226 = case shown="True" w321 {
          tunnel: w320 -> [_ w327]
          frame False {
          }
          frame True {
            n227 = local read "List of devices"() -> (w332:T3)
            n228 = local read "Device"() -> (w331:u16)
            n229 = Index Array(array=w332, index=w331) -> (element=w330:T4)
            n230 = Unbundle By Name(w330) -> ("List of locations"=w329:T2[])
            n231 = Array Size(array=w329) -> (size(s)=w324:i32)
            n232 = In Range and Coerce(upper limit=w324, x=w327, lower limit=0) -> (coerced(x)=w325:i32, In Range?=w326:bool)
            n233 = case shown="True" w326 {
              tunnel: w329 -> [_ w335]
              tunnel: w325 -> [_ w334]
              frame False {
              }
              frame True {
                n234 = Index Array(array=w335, index=w334) -> (element=w333:T2)
                n235 = property on="Goto Location" class="Clust (strict)"("Val(Sgnl)"=w333) -> ()  [unwired: 2 in, 2 out]
              }
            }
          }
        }
      }
      event "Add location": Value Change {
        n236 = event-data() -> ("NewVal"=w339:bool)  [unwired: 1 in, 5 out]
        n237 = case shown="True" w339 {
          tunnel: [_ FALSE ("Add location")] -> w338
          frame False {
          }
          frame True {
            w342 = u16 0 items=["Add/set", "Delete"] ("Function")
            n238 = local read "Current Location"() -> (w340:T2)
            n239 = local read "List of devices"() -> (w346:T3)
            n240 = local read "List of default devices"() -> (w344:T3)
            n241 = local read "Device"() -> (w341:u16)
            n242 = call "add or delete location.vi"("Function"=w342, "List of defaults"=w344, "New location"=w340, "Device in"=w341, "List of devices in"=w346) -> ("List of devices out"=w343:T3)  [unwired: 4 in, 2 out]
            n243 = property on="List of devices" class="Arr (strict)"("Val(Sgnl)"=w343) -> ()  [unwired: 2 in, 2 out]
          }
        }
        n244 = local write "Add location"(w338) -> ()
      }
      event "Delete device": Value Change {
        n245 = event-data() -> ("NewVal"=w348:bool)  [unwired: 1 in, 5 out]
        n246 = case shown="True" w348 {
          tunnel: [_ FALSE ("Delete device")] -> w347
          frame False {
          }
          frame True {
            w349 = u16 1 items=["Add/set", "Delete"] ("Function")
            n247 = local read "List of devices"() -> (w352:T3)
            n248 = local read "Device"() -> (w350:u16)
            n249 = call "add or delete location.vi"("Function"=w349, "Device in"=w350, "List of devices in"=w352) -> ("List of devices out"=w351:T3)  [unwired: 6 in, 2 out]
            n250 = property on="List of devices" class="Arr (strict)"("Val(Sgnl)"=w351) -> ()  [unwired: 2 in, 2 out]
          }
        }
        n251 = local write "Delete device"(w347) -> ()
      }
      event "Save device list": Value Change {
        n252 = event-data() -> ("NewVal"=w355:bool)  [unwired: 1 in, 5 out]
        n253 = case shown="True" w355 {
          tunnel: [_ FALSE ("Save device list")] -> w354
          frame False {
          }
          frame True {
            n254 = local read "Default File Path"() -> (w356:path)
            n255 = call "File Dialog"("start path"=w356) -> ("selected path"=w358:path, "error out"=w357:errorcluster)  [unwired: 11 in, 2 out]
            n256 = case shown="No Error" w357 {
              tunnel: w358 -> [w366 _]
              frame No Error {
                w360 = u16 1 items=["Load", "Save"] ("Mode")
                n257 = local read "List of devices"() -> (w363:T3)
                n258 = local read "List of default devices"() -> (w362:T3)
                n259 = call "load or save device list.vi"("Type"="Device", "Mode"=w360, "selected path"=w366, "List of devices in"=w363) -> ("file path out"=w364:path)  [unwired: 6 in, 1 out]
                n260 = call "load or save device list.vi"("Type"="Default", "Mode"=w360, "selected path"=w364, "List of devices in"=w362) -> ()  [unwired: 6 in, 2 out]
              }
              frame Error {
              }
            }
          }
        }
        n261 = local write "Save device list"(w354) -> ()
      }
      event "Load device list": Value Change {
        n262 = event-data() -> ("NewVal"=w368:bool)  [unwired: 1 in, 5 out]
        n263 = case shown="True" w368 {
          tunnel: [_ FALSE ("Load device list")] -> w367
          frame False {
          }
          frame True {
            n264 = local read "Default File Path"() -> (w371:path)
            n265 = call "File Dialog2"("start path"=w371) -> ("selected path"=w369:path, "error out"=w370:errorcluster)  [unwired: 11 in, 2 out]
            n266 = case shown="No Error" w370 {
              tunnel: w369 -> [w379 _]
              frame No Error {
                w375 = u16 0 items=["Load", "Save"] ("Mode")
                n267 = call "load or save device list.vi"("Type"="Device", "Mode"=w375, "selected path"=w379) -> ("file path out"=w376:path, "List of devices out"=w378:T3)  [unwired: 7 in]
                n268 = property on="List of devices" class="Arr (strict)"("Val(Sgnl)"=w378) -> ()  [unwired: 2 in, 2 out]
                n269 = call "load or save device list.vi"("Type"="Default", "Mode"=w375, "selected path"=w376) -> ("List of devices out"=w374:T3)  [unwired: 7 in, 1 out]
                n270 = local write "List of default devices"(w374) -> ()
              }
              frame Error {
              }
            }
          }
        }
        n271 = local write "Load device list"(w367) -> ()
      }
      event Value Change {
        n272 = event-data() -> ("NewVal"=w385:T3)  [unwired: 1 in, 5 out]
        n273 = for {
          tunnel: w385 -> [w398] mode=indexing
          shift-right: [w395] -> w392
          shift-left: T7 [] ("Annotation List") -> [w396]
          tunnel: [w394] -> w391 mode=indexing
          n274 = Unbundle By Name(w398) -> ("Device Description"=w394:string, "List of locations"=w397:T2[])
          n275 = for {
            tunnel: w397 -> [w409] mode=indexing
            tunnel: w394 -> [w405]
            shift-right: [w400] -> w395
            shift-left: w396 -> [w402]
            n276 = Unbundle By Name(w409) -> ("Description"=w407:string, "Position"=w408:cluster{"Position X":dbl, "Position Y":dbl})
            n277 = Concatenate Strings(w405, "\r", w407) -> (w404:string)
            n278 = Bundle By Name(cluster=T8 {"Name"="", "Color"=16776960, "Style"=4, "Point Style"=13, "Name Visible"=TRUE, "Allow Drag"=FALSE, "Annotation Mode"=0, "Plot"=-1, "Index"=0, "Position"={"X"=0.0, "Y"=0.0}, "X Scale"=0, "Y Scale"=0, "Show Arrow"=FALSE, "Lock Name"=FALSE, "Plot Area"=0, "Label Offset"={"X"=0.0, "Y"=0.0}} ("element"), "Name"=w404, "Position"=w408, "Color"=u32 16448250) -> (w401:T8)
            n279 = Insert Into Array(array=w402, new element=w401) -> (w400:T7)  [unwired: 1 in]
          }
        }
        n280 = property on="Device" class="Ring (strict)"("Strings []"=w391) -> ("NumItems"=w387:u32, "Value"=w390:u16)  [unwired: 2 in, 2 out]
        n281 = property on="Location plot" class="XYGraph (strict)"("AnntList"=w392) -> ()  [unwired: 2 in, 2 out]
        n282 = Decrement(x=w387) -> (x-1=w386:u32)
        n283 = In Range and Coerce(upper limit=w386, x=w390, lower limit=u32 0) -> (coerced(x)=w388:u32)  [unwired: 1 out]
        n284 = local read "Radius Limit (mm)"() -> (w380:dbl)
        n285 = property on="Device" class="Ring (strict)"("Val(Sgnl)"=w388) -> ()  [unwired: 2 in, 2 out]
        n286 = call "generate limit circle.vi"("Radius Limit (mm)"=w380, "Location Description"="Location Description", "NewVal"=w385, "Device Description"="Device Description") -> ("Center location"=→"Center location":T2, "Circle"=→"Circle":cluster{dbl[], dbl[]})  [unwired: 6 in]
      }
      event "Device": Value Change {
        n287 = event-data() -> ("NewVal"=w414:u16)  [unwired: 1 in, 5 out]
        n288 = local read "List of devices"() -> (w415:T3)
        n289 = Index Array(array=w415, index=w414) -> (element=w413:T4)
        n290 = property on="nSWAT quick move diagram" class="Clust (strict)"() -> ("Controls[]"=w411:refnum<vi>[])  [unwired: 2 in, 2 out]
        n291 = Unbundle By Name(w413) -> ("List of locations"=w412:T2[])
        n292 = for {
          tunnel: w411 -> [w418] mode=indexing
          tunnel: [w416] -> w410 mode=indexing
          w419 = refnum<vi> refnum  # Boolean
          n293 = To More Specific Class(target class=w419, reference=w418) -> (specific class reference=w420:refnum<vi>)  [unwired: 1 in, 1 out]
          n294 = property class="Bool"(reference=w420, "BoolText.Text"="" ("Boolean Text.Text")) -> (reference out=w416:refnum<vi>)  [unwired: 1 in, 1 out]
        }
        n295 = for {
          tunnel: w412 -> [w422] mode=indexing
          tunnel: w410 -> [w424] mode=indexing
          w425 = refnum<vi> refnum  # Boolean
          n296 = Unbundle By Name(w422) -> ("Description"=w421:string)
          n297 = To More Specific Class(target class=w425, reference=w424) -> (specific class reference=w423:refnum<vi>)  [unwired: 1 in, 1 out]
          n298 = property class="Bool"(reference=w423, "BoolText.Text"=w421) -> ()  [unwired: 1 in, 2 out]
        }
      }
      event "Location plot": Mouse Down? {
        n299 = event-data() -> ("Coords"=w429:T9, "Button"=w428:u16)  [unwired: 1 in, 6 out]
        n300 = property on="Location plot" class="XYGraph (strict)"() -> ("ActPaletteTool"=w427:i32)  [unwired: 2 in, 2 out]
        n301 = case shown="1" w428 {
          tunnel: w429 -> [_ w431 _]
          tunnel: w427 -> [_ w430 w462]
          tunnel: [_ _ w461] -> w426
          frame 0, Default {
          }
          frame 1 {
            n302 = case shown="0" w430 {
              tunnel: w431 -> [w454 _]
              frame 0 {
                n303 = local read "Mouse over item?"() -> (w448:bool)
                n304 = case shown="False" w448 {
                  tunnel: w454 -> [w456 _]
                  tunnel: [w455 w457] -> w449
                  frame False {
                    n305 = invoke on="Location plot" class="XYGraph (strict)" method="Map Coords To XY"("Coords"=w456) -> ("XY"=w455:cluster{"X":dbl, "Y":dbl})  [unwired: 6 in, 6 out]
                  }
                  frame True {
                    n306 = local read "Mouse over location"() -> (w457:cluster{"X":dbl, "Y":dbl})
                  }
                }
                n307 = local read "Center location"() -> (w447:T2)
                n308 = Unbundle By Name(w447) -> ("Position.Position X"=w445:dbl, "Position.Position Y"=w443:dbl)
                n309 = property on="Location plot" class="XYGraph (strict)"() -> ("XScale.Maximum"=w453:dbl, "XScale.Minimum"=w452:dbl, "YScale.Maximum"=w451:dbl, "YScale.Minimum"=w450:dbl)  [unwired: 2 in, 2 out]
                n310 = Unbundle By Name(w449) -> ("X"=w446:dbl, "Y"=w444:dbl)
                n311 = Subtract(x=w446, y=w445) -> (x-y=w442:dbl)
                n312 = Subtract(x=w444, y=w443) -> (x-y=w441:dbl)
                n313 = In Range and Coerce(upper limit=w451, x=w444, lower limit=w450) -> (In Range?=w434:bool)  [unwired: 1 out]
                n314 = In Range and Coerce(upper limit=w453, x=w446, lower limit=w452) -> (In Range?=w435:bool)  [unwired: 1 out]
                n315 = local read "Radius Limit (mm)"() -> (w436:dbl)
                n316 = Square(x=w442) -> (x^2=w440:dbl)
                n317 = Square(x=w441) -> (x^2=w439:dbl)
                n318 = Add(x=w440, y=w439) -> (x+y=w438:dbl)
                n319 = Square Root(x=w438) -> (sqrt(x)=w437:dbl)
                n320 = Less?(x=w437, y=w436) -> (x < y?=w433:bool)
                n321 = Compound Arithmetic op=AND(w435, w434, w433) -> (w432:bool)
                n322 = case shown="True" w432 {
                  tunnel: w449 -> [_ w458]
                  frame False {
                  }
                  frame True {
                    n323 = Bundle By Name(cluster=T2 {"Description"="", "Position"={"Position X"=0.0, "Position Y"=0.0}} ("Value (Signaling)"), "Position"=w458) -> (w460:T2)
                    n324 = property on="Last click location" class="Clust (strict)"("Value"=w458) -> ()  [unwired: 2 in, 2 out]
                    n325 = property on="Goto Location" class="Clust (strict)"("Val(Sgnl)"=w460) -> ()  [unwired: 2 in, 2 out]
                  }
                }
              }
              frame 1, Default {
              }
            }
          }
          frame 2 {
            n326 = case shown="0" w462 {
              tunnel: [w463 _] -> w461
              frame 0 {
                n327 = local read "Mouse over item?"() -> (w464:bool)
                n328 = case shown="True" w464 {
                  tunnel: [_ TRUE ("Discard?")] -> w463
                  frame False {
                  }
                  frame True {
                    n329 = local read "Mouse over location"() -> (w470:cluster{"X":dbl, "Y":dbl})
                    n330 = local read "List of devices"() -> (w469:T3)
                    n331 = for {
                      tunnel: w469 -> [w481] mode=indexing
                      tunnel: w470 -> [w479]
                      tunnel: [w478] -> w468
                      tunnel: [w477] -> w467
                      tunnel: [w476] -> w466
                      i -> [w476]
                      stop <- w478 stop-if-true
                      n332 = Unbundle By Name(w481) -> ("List of locations"=w480:T2[])
                      n333 = for {
                        tunnel: w480 -> [w488] mode=indexing
                        tunnel: w479 -> [w487]
                        tunnel: [w483] -> w478
                        tunnel: [w482] -> w477
                        i -> [w482]
                        stop <- w483 stop-if-true
                        n334 = Unbundle By Name(w488) -> ("Position"=w486:cluster{"Position X":dbl, "Position Y":dbl})
                        n335 = Equal?(x=w487, y=w486) -> (x = y?=w485:cluster{bool, bool})
                        n336 = Cluster To Array(cluster=w485) -> (array=w484:bool[])
                        n337 = And Array Elements(Boolean array=w484) -> (logical AND=w483:bool)
                      }
                    }
                    n338 = case shown="True" w468 {
                      tunnel: w469 -> [_ w475]
                      tunnel: w467 -> [_ w474]
                      tunnel: w466 -> [_ w473]
                      frame False {
                      }
                      frame True {
                        w472 = u16 1 items=["Add/set", "Delete"] ("Function")
                        n339 = call "add or delete location.vi"("Function"=w472, "Location in"=w474, "Device in"=w473, "List of devices in"=w475) -> ("List of devices out"=w471:T3)  [unwired: 5 in, 2 out]
                        n340 = property on="List of devices" class="Arr (strict)"("Val(Sgnl)"=w471) -> ()  [unwired: 2 in, 2 out]
                      }
                    }
                  }
                }
              }
              frame 1, Default {
              }
            }
          }
        }
        n341 = event-data("Discard?"=w426) -> ()  [unwired: 1 in, 1 out]
      }
      event "Location plot": Mouse Move {
        n342 = event-data() -> ("Coords"=w490:T9)  [unwired: 1 in, 4 out]
        n343 = property on="Location plot" class="XYGraph (strict)"() -> ("ActPaletteTool"=w489:i32)  [unwired: 2 in, 2 out]
        n344 = case shown="0, Default" w489 {
          tunnel: w490 -> [w503 _]
          frame 0, Default {
            n345 = property on="Location plot" class="XYGraph (strict)"() -> ("XScale.Maximum"=w501:dbl, "XScale.Minimum"=w500:dbl)  [unwired: 2 in, 2 out]
            n346 = property on="Location plot" class="XYGraph (strict)"() -> ("AnntList"=w491:T7)  [unwired: 2 in, 2 out]
            n347 = invoke on="Location plot" class="XYGraph (strict)" method="Map Coords To XY"("Coords"=w503) -> ("XY"=w502:cluster{"X":dbl, "Y":dbl})  [unwired: 6 in, 6 out]
            n348 = Subtract(x=w501, y=w500) -> (x-y=w499:dbl)
            n349 = Absolute Value(x=w499) -> (abs(x)=w497:dbl)
            n350 = Divide(x=w497, y=55.0) -> (x/y=w494:dbl)
            n351 = Bundle(w494, w494) -> (w498:cluster{dbl, dbl})  [unwired: 1 in]
            n352 = for {
              tunnel: w491 -> [w516] mode=indexing
              tunnel: w502 -> [w518]
              tunnel: [w505] -> w493 mode=indexing
              tunnel: w498 -> [w517]
              tunnel: [w515] -> w495 mode=indexing
              n353 = Unbundle By Name(w516) -> ("Position"=w504:cluster{"X":dbl, "Y":dbl})  [unwired: 1 out]
              n354 = Add(x=w518, y=w517) -> (x+y=w511:cluster{dbl, dbl})
              n355 = Subtract(x=w518, y=w517) -> (x-y=w510:cluster{dbl, dbl})
              n356 = Less?(x=w504, y=w511) -> (x < y?=w509:cluster{bool, bool})
              n357 = Greater?(x=w504, y=w510) -> (0:w508:cluster{bool, bool})
              n358 = And(x=w509, y=w508) -> (x .and. y?=w507:cluster{bool, bool})
              n359 = Cluster To Array(cluster=w507) -> (array=w506:bool[])
              n360 = And Array Elements(Boolean array=w506) -> (logical AND=w505:bool)
              n361 = Select(t=u32 6618880, s=w505, f=u32 16448250) -> (s? t:f=w513:u32)
              n362 = Bundle By Name(cluster=w516, "Color"=w513) -> (w515:T8)
              n363 = case shown="True" w505 {
                tunnel: w504 -> [_ w519]
                frame False {
                }
                frame True {
                  "Mouse over location" <- w519
                }
              }
            }
            n364 = Or Array Elements(Boolean array=w493) -> (logical OR=→"Mouse over item?":bool)
            n365 = property on="Location plot" class="XYGraph (strict)"("AnntList"=w495) -> ()  [unwired: 2 in, 2 out]
          }
          frame 1 {
          }
        }
      }
      event "Location plot": Mouse Wheel {
        n366 = event-data() -> ("Coords"=w540:T9, "Delta"=w544:i32)  [unwired: 1 in, 8 out]
        n367 = Greater Than 0?(x=w544) -> (x > 0?=w543:bool)
        n368 = invoke on="Location plot" class="XYGraph (strict)" method="Map Coords To XY"("Coords"=w540) -> ("XY"=w539:cluster{"X":dbl, "Y":dbl})  [unwired: 6 in, 6 out]
        n369 = Select(t=0.8, s=w543, f=1.2) -> (s? t:f=w520:dbl)
        n370 = property on="Location plot" class="XYGraph (strict)"() -> ("XScale.Maximum"=w529:dbl, "XScale.Minimum"=w538:dbl, "YScale.Maximum"=w523:dbl, "YScale.Minimum"=w532:dbl)  [unwired: 2 in, 2 out]
        n371 = Unbundle By Name(w539) -> ("X"=w528:dbl, "Y"=w522:dbl)
        n372 = Subtract(x=w528, y=w538) -> (x-y=w537:dbl)
        n373 = Subtract(x=w529, y=w528) -> (x-y=w530:dbl)
        n374 = Subtract(x=w522, y=w532) -> (x-y=w533:dbl)
        n375 = Subtract(x=w523, y=w522) -> (x-y=w524:dbl)
        n376 = Multiply(x=w537, y=w520) -> (x*y=w536:dbl)
        n377 = Multiply(x=w530, y=w520) -> (x*y=w527:dbl)
        n378 = Multiply(x=w533, y=w520) -> (x*y=w534:dbl)
        n379 = Multiply(x=w524, y=w520) -> (x*y=w525:dbl)
        n380 = Subtract(x=w528, y=w536) -> (x-y=w535:dbl)
        n381 = Subtract(x=w522, y=w534) -> (x-y=w531:dbl)
        n382 = Add(x=w528, y=w527) -> (x+y=w526:dbl)
        n383 = Add(x=w522, y=w525) -> (x+y=w521:dbl)
        n384 = property on="Location plot" class="XYGraph (strict)"("XScale.Maximum"=w526, "XScale.Minimum"=w535, "YScale.Maximum"=w521, "YScale.Minimum"=w531) -> ()  [unwired: 2 in, 2 out]
      }
      event "Rescale location plot": Value Change {
        n385 = event-data() -> ("NewVal"=w546:bool)  [unwired: 1 in, 5 out]
        n386 = case shown="True" w546 {
          tunnel: [_ FALSE ("Rescale location plot")] -> w545
          frame False {
          }
          frame True {
            w564 = 10.0 ("y")
            w563 = 10.0 ("y")
            # "range"
            n387 = property on="Location plot" class="XYGraph (strict)"() -> ("AnntList"=w588:T7)  [unwired: 2 in, 2 out]
            n388 = local read "Circle"() -> (w553:cluster{dbl[], dbl[]})
            n389 = for {
              tunnel: w588 -> [w592] mode=indexing
              tunnel: [w591] -> w552 mode=indexing
              tunnel: [w590] -> w550 mode=indexing
              n390 = Unbundle By Name(w592) -> ("Position.X"=w591:dbl, "Position.Y"=w590:dbl)
            }
            n391 = Unbundle(w553) -> (w551:dbl[], w549:dbl[])
            n392 = Build Array (concatenate)(w550, w549) -> (w547:dbl[])
            n393 = Build Array (concatenate)(w552, w551) -> (w548:dbl[])
            n394 = Array Max & Min(array=w547) -> (max value=w586:dbl, min value=w581:dbl)  [unwired: 2 out]
            n395 = Array Max & Min(array=w548) -> (max value=w587:dbl, min value=w554:dbl)  [unwired: 2 out]
            n396 = Subtract(x=w587, y=w554) -> (x-y=w577:dbl)
            n397 = Subtract(x=w586, y=w581) -> (x-y=w583:dbl)
            n398 = Greater?(x=w577, y=w583) -> (0:w585:bool)
            n399 = Select(t=w577, s=w585, f=w583) -> (s? t:f=w584:dbl)
            n400 = Multiply(x=w584, y=12.0) -> (x*y=w576:dbl)
            n401 = Round Toward +Infinity(x=w576) -> (ceil(x): smallest int >= x=w575:dbl)
            n402 = Divide(x=w575, y=10.0) -> (x/y=w568:dbl)
            n403 = In Range and Coerce(upper limit=1000.0, x=w568, lower limit=1.0) -> (coerced(x)=w567:dbl)  [unwired: 1 out]
            n404 = Subtract(x=w567, y=w577) -> (x-y=w578:dbl)
            n405 = Divide(x=w578, y=2.0) -> (x/y=w579:dbl)
            n406 = Subtract(x=w554, y=w579) -> (x-y=w574:dbl)
            n407 = Subtract(x=w567, y=w583) -> (x-y=w582:dbl)
            n408 = Multiply(x=w574, y=w563) -> (x*y=w573:dbl)
            n409 = Divide(x=w582, y=2.0) -> (x/y=w580:dbl)
            n410 = Round Toward -Infinity(1:w573) -> (0:w572:dbl)
            n411 = Divide(x=w572, y=w563) -> (x/y=w555:dbl)
            n412 = Subtract(x=w581, y=w580) -> (x-y=w569:dbl)
            n413 = Multiply(x=w569, y=w564) -> (x*y=w570:dbl)
            n414 = Add(x=w555, y=w567) -> (x+y=w557:dbl)
            n415 = Round Toward -Infinity(1:w570) -> (0:w571:dbl)
            n416 = Divide(x=w571, y=w564) -> (x/y=w558:dbl)
            n417 = Add(x=w558, y=w567) -> (x+y=w556:dbl)
            n418 = property on="Location plot" class="XYGraph (strict)"("XScale.Maximum"=w557, "XScale.Minimum"=w555, "YScale.Maximum"=w556, "YScale.Minimum"=w558) -> ()  [unwired: 2 in, 2 out]
          }
        }
        n419 = local write "Rescale location plot"(w545) -> ()
      }
      event "Radius Limit (mm)": Value Change {
        n420 = event-data() -> ()  [unwired: 1 in, 6 out]
        n421 = local read "List of devices"() -> (w593:T3)
        n422 = property on="List of devices" class="Arr (strict)"("Val(Sgnl)"=w593) -> ()  [unwired: 2 in, 2 out]
      }
    }
  }
  n423 = Unregister For Events(event registration refnum=w10, error in=w4) -> (error out=w7:errorcluster)
  n424 = call <vilib>:"Cancel Value Change Notifications.vi"("error in (no error)"=w7, "shared variables"=w2, "notification refnum"=w6) -> ("error out"=w9:errorcluster, "shared variable value change notification"=w8:refnum<user-event>)  [unwired: 6 in, 1 out]
  n425 = call <vilib>:"Disable Value Change Notifications.vi"("error in (no error)"=w9, "notification refnum"=w8) -> ()  [unwired: 9 in, 1 out]
  n426 = for {
    N: w17 -> [_]
    tunnel: [w594] -> w19 mode=indexing
    i -> [w594]
  }
  n427 = Divide(x=w19, y=w17) -> (x/y=w20:dbl[])
  n428 = local read "Radius Limit (mm)"() -> (w24:dbl)
  n429 = Multiply(x=w20, y=6.283185307179586) -> (x*y=w21:dbl[])
  n430 = Cosine(x=w21) -> (cos(x)=w22:dbl[])
  n431 = Sine(x=w21) -> (sin(x)=w23:dbl[])
  n432 = Multiply(x=w22, y=w24) -> ()  [unwired: 1 out]
  n433 = Multiply(x=w23, y=w24) -> ()  [unwired: 1 out]
